vi "TDMS to ASCII Convert Service.vi"() -> ()   [LabVIEW 2010, in "TDMS to ASCII Convert.lvlib"]
uses:
  TDMS to ASCII Convert.lvlib
  Stop FGV Commands.ctl
  <vilib>/NI Veristand/Execution/Stimulus/StimulusState.ctl
  Queue Typedef.ctl
  <vilib>/NI Veristand/Execution/Stimulus/NI_VS Stimulus ExecutionAPI.lvlib
  <vilib>/ptbypt/NI_PtbyPt.lvlib
panel:
  in  "NIVS.Workspace Event":refnum<event-registration>
  in  "NIVS.Project File Path":path
  in  "NIVS.Gateway IP Address":string
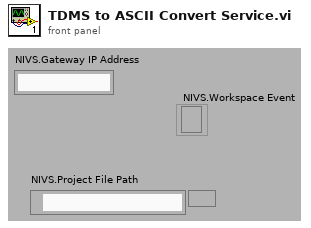
[diagram p1: front panel]
types:
  T1 = typedef "TDMS to ASCII Convert.lvlib/Service Ref Cluster.ctl" = cluster{"queue":refnum<queue>, "Workspace":T2, "Stim":T3, "Events":cluster{"SystemChangeEventRef":T4, "NIVS.Workspace Event":refnum<event-registration>}, "SystemStateRefs":T5, "Logs folder":path}
  T2 = typedef "NI_VS Workspace ExecutionAPI.lvlib/WorkspaceAPI.ctl" = refnum<k24>
  T3 = typedef "NI_VS Stimulus ExecutionAPI.lvlib/StimulusAPI.ctl" = refnum<k24>
  T4 = typedef "NI_VS Workspace ExecutionAPI.lvlib/SystemStateRegEventRef.ctl" = refnum<event-registration>
  T5 = typedef "NI_VS Workspace ExecutionAPI.lvlib/SystemStateEventRef.ctl" = cluster{"CustDatRef":refnum<user-event>, "EvtRef":refnum<k27>}
  T6 = cluster{"SystemChangeEventRef":T4, "NIVS.Workspace Event":refnum<event-registration>}
  T7 = typedef "TDMS to ASCII Convert.lvlib/Stop FGV Commands.ctl" = enum16{"Write", "Read", "Reset"}
  T8 = typedef "NI_VS Stimulus ExecutionAPI.lvlib/StimulusState.ctl" = enum16{"Stopped", "Starting", "Running", "Stopping"}
  T9 = typedef "TDMS to ASCII Convert.lvlib/Queue Typedef.ctl" = cluster{"Path":path, "TDMS Logs":path[]}
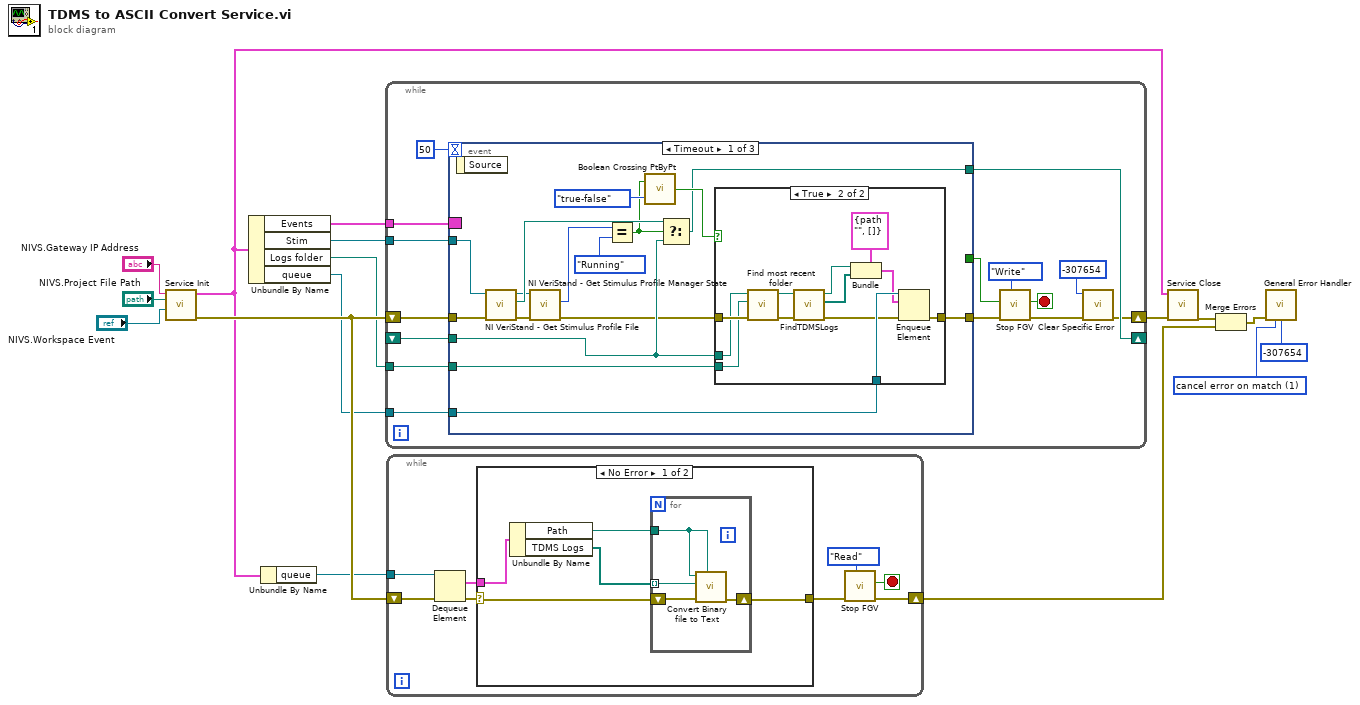
[diagram p0: block diagram]
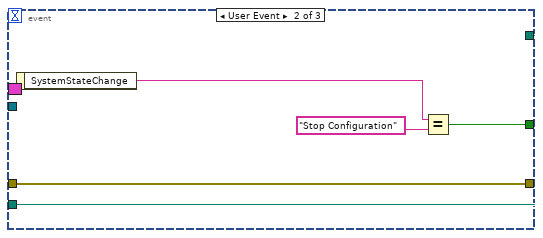
[diagram p3: hidden frame]
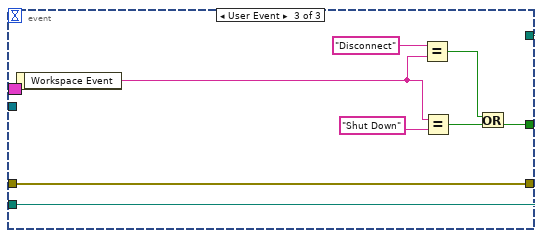
[diagram p4: hidden frame]
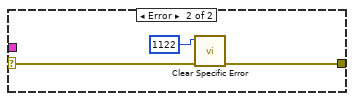
[diagram p5: hidden frame]
diagram:
  w13 = 1 items=["no exception", "cancel error on match", "set error on match"] ("[exception action] (none:0)")
  n1 = call "Service Init.vi"("NIVS.Workspace Event"="NIVS.Workspace Event", "NIVS.Project File Path"="NIVS.Project File Path", "NIVS.Gateway IP Address"="NIVS.Gateway IP Address") -> ("error out"=w14:errorcluster, "System Refs Cluster"=w11:T1)  [unwired: 7 in]
  n2 = Unbundle By Name(w11) -> ("Events"=w4:T6, "Stim"=w8:T3, "Logs folder"=w7:path, "queue"=w6:refnum<queue>)
  n3 = Unbundle By Name(w11) -> ("queue"=w5:refnum<queue>)
  n4 = while {
    shift-right: [w29] -> _
    shift-left: _ -> [w28]
    shift-right: [w17] -> w3
    shift-left: w14 -> [w31]
    tunnel: w8 -> [w25]
    tunnel: w7 -> [w24]
    tunnel: w6 -> [w23]
    tunnel: w4 -> [w22]
    stop <- w21 stop-if-true
    n5 = event shown="[0] Timeout" {
      selector: w22 -> [_ _ _]
      dyn-events: _ -> [_ _ _]
      timeout: 50 -> [_ _ _]
      tunnel: [w32 w65 w73] -> w20
      tunnel: w31 -> [w39 w65 w73]
      tunnel: [_ w63 w67] -> w26
      tunnel: [w43 w62 w71] -> w29
      tunnel: w28 -> [w42 w62 w71]
      tunnel: w25 -> [w35 _ _]
      tunnel: w24 -> [w34 _ _]
      tunnel: w23 -> [w33 _ _]
      event Timeout {
        n6 = event-data() -> ()  [unwired: 1 in, 1 out]
        n7 = call <vilib>:"NI VeriStand - Get Stimulus Profile File.vi"("error in (no error)"=w39, "StimulusProfileManager in"=w35) -> ("error out"=w38:errorcluster, "File"=w41:path, "StimulusProfileManager out"=w36:T3)  [unwired: 7 in]
        n8 = call <vilib>:"NI VeriStand - Get Stimulus Profile Manager State.vi"("error in (no error)"=w38, "StimulusProfileManager in"=w36) -> ("error out"=w37:errorcluster, "State"=w47:T8)  [unwired: 7 in, 1 out]
        n9 = Equal?(x=w47, y=StimulusState."Running") -> (x = y?=w40:bool)
        n10 = call <vilib>:"Boolean Crossing PtByPt.vi"("direction"=enum16{"either", "false-true", "true-false"}."true-false", "input"=w40) -> ("crossing"=w44:bool)  [unwired: 1 in]
        n11 = Select(t=w41, s=w40, f=w42) -> (s? t:f=w43:path)
        n12 = case shown="True" w44 {
          tunnel: w37 -> [w48 w60]
          tunnel: [w48 w58] -> w32
          tunnel: w42 -> [_ w57]
          tunnel: w34 -> [_ w56]
          tunnel: w33 -> [_ w59]
          frame False {
          }
          frame True {
            n13 = call "Find most recent folder.vi"("error in (no error)"=w60, "Directory to search"=w56, "File path (used for pattern search)"=w57) -> ("error out"=w53:errorcluster, "most recent folder"=w52:path)  [unwired: 7 in]
            n14 = call "FindTDMSLogs.vi"("error in (no error)"=w53, "Directory to search"=w52) -> ("error out"=w49:errorcluster, "TDMS Files"=w50:path[], "Directory to search out"=w51:path)  [unwired: 7 in]
            n15 = Bundle(cluster=T9 {"Path"=path "", "TDMS Logs"=[]} ("Queue Data"), "Path"=w51, "TDMS Logs"=w50) -> (w54:T9)
            n16 = Enqueue Element(queue=w59, element=w54, error in (no error)=w49) -> (error out=w58:errorcluster)  [unwired: 1 in, 2 out]
          }
        }
      }
      event User Event {
        n17 = event-data() -> ("SystemStateChange"=w64:string)  [unwired: 1 in]
        n18 = Equal?(x=w64, y="Stop Configuration" ("x")) -> (x = y?=w63:bool)
      }
      event User Event {
        n19 = event-data() -> ("Workspace Event"=w69:string)  [unwired: 1 in]
        n20 = Equal?(x="Disconnect", y=w69) -> (x = y?=w66:bool)
        n21 = Equal?(x=w69, y="Shut Down" ("x")) -> (x = y?=w72:bool)
        n22 = Or(x=w66, y=w72) -> (x .or. y?=w67:bool)
      }
    }
    n23 = call "Stop FGV.vi"("Command"=Stop_FGV_Commands."Write", "error in (no error)"=w20, "Stop?"=w26) -> ("error out"=w18:errorcluster, "Latched Stop"=w21:bool)  [unwired: 6 in, 1 out]
    n24 = call "Clear Specific Error.vi"("error in (no error)"=w18, "code"=-307654 ("y")) -> ("error out"=w17:errorcluster)  [unwired: 9 in]
  }
  n25 = while {
    shift-right: [w79] -> w1
    shift-left: w14 -> [w81]
    tunnel: w5 -> [w76]
    stop <- w75 stop-if-true
    n26 = Dequeue Element(queue=w76, error in (no error)=w81) -> (element=w77:T9, error out=w80:errorcluster)  [unwired: 1 in, 2 out]
    n27 = case shown="No Error" w80 {
      selector: w80 -> [w82 w91]
      tunnel: [w86 w93] -> w74
      tunnel: w77 -> [w85 _]
      frame No Error {
        n28 = Unbundle By Name(w85) -> ("Path"=w84:path, "TDMS Logs"=w83:path[])
        n29 = for {
          shift-right: [w89] -> w86
          shift-left: w82 -> [w90]
          tunnel: w84 -> [w88]
          tunnel: w83 -> [w87] mode=indexing
          n30 = call "Convert Binary file to Text.vi"("Originating directory"=w88, "error in (no error)"=w90, "TDMS File Path"=w87, "Destination directory"=w88) -> ("error out"=w89:errorcluster)  [unwired: 7 in]
        }
      }
      frame Error {
        n31 = call "Clear Specific Error.vi"("error in (no error)"=w91, "code"=1122 ("y")) -> ("error out"=w93:errorcluster)  [unwired: 9 in]
      }
    }
    n32 = call "Stop FGV.vi"("Command"=Stop_FGV_Commands."Read", "error in (no error)"=w74) -> ("error out"=w79:errorcluster, "Latched Stop"=w75:bool)  [unwired: 7 in, 1 out]
  }
  n33 = call "Service Close.vi"("error in (no error)"=w3, "Service Refs Cluster"=w11) -> ("error out"=w2:errorcluster)  [unwired: 9 in]
  n34 = Merge Errors(w2, w1) -> (w10:errorcluster)
  n35 = call <vilib>:"General Error Handler.vi"("error in (no error)"=w10, "[exception action] (none:0)"=w13, "[exception code]"=-307654) -> ()  [unwired: 8 in, 5 out]
